vi "Property_Tree Tag_Encode.vi"(7 "Action":T2, 8 "Class":string, 9 "Property Type":T1(ring), 10 "Index":u16, 11 "Method/Property Info":T3) -> (0 "Parents":string[](array[string]), 1 "Indent":i32, 2 "Tag":string, 3 "Bare name":string, 5 "Full name":string)   [LabVIEW 2023]
doc: "By using the long name localized for the tag, children of search matches will be shown. ID is required in tag bc we set the property node terminals by ID.\n\nThe display valule will be the short name for property and method dialogs, and the full name for remove and rearrange dialongs.\n\nFormat is\n\nindex,propertyType,Class,[classID.]ID sting,[class.]parent:shortName \n\nwhere parent:shortName=Long name (localized)\nclass=class of the childmost class in list\nfor dotted properties, the ID string will be of the form classID.propertyID, and the Display name will be of the form Label.Property. \n\nConsider The dotted property Caption.Font. Caption has the class type of Text, so the Class for this tag will be Text, the class ID is 5, and the label contains the Property name \"caption\""
uses:
  controls/action enum.ctl
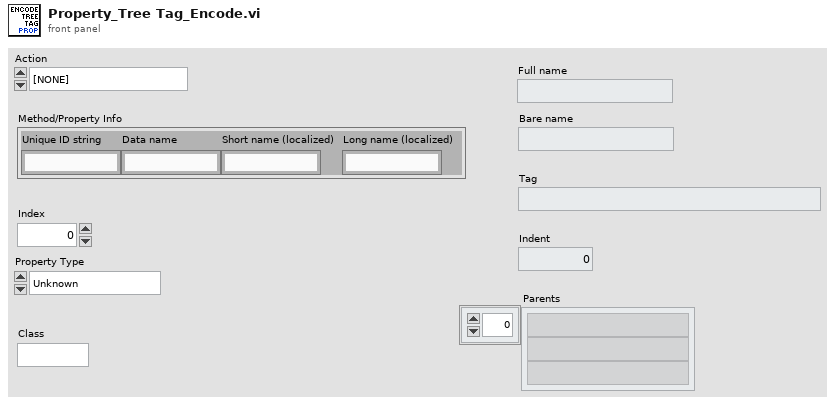
[diagram p1: front panel]
types:
  T1 = enum16{"Unknown", "Base", "Scripting", "Private", "Deprecated", "None", "Divider"}
  T2 = typedef "action enum.ctl" = enum16{"[NONE]", "Wire Bundle", "Wire Unbundle", "Terminal Unbundle", "Terminal Bundle", "Bundler Move Up", "Bundler Move Down", "Bundler Insert", "Bundler Remove", "Bundler Remove Unwired", "Bundler Rearrange", "In Place Insert", "In Place Remove", "In Place Remove Unwired", "In Place Rearrange", "Wire Properties", "Wire Method", "Terminal Properties", "Terminal Method", "Property Move Up", "Property Move Down", "Properties Insert", "Properties Remove", "Properties Remove Unwired", "Properties Rearrange", "Method Change", "Class for Constant", "Class For Control", "Class For Node", "Class Name to Clipboard"}
  T3 = cluster{"Unique ID string":string, "Data name":string, "Short name (localized)":string, "Long name (localized)":string}
  T4 = cluster{"Undotted Property":string, "Bare Property":string, "Is dotted?":bool, "Dot depth":i32, "Indent":i32, "Property Hierarchy":string[], "Parents":string[]}
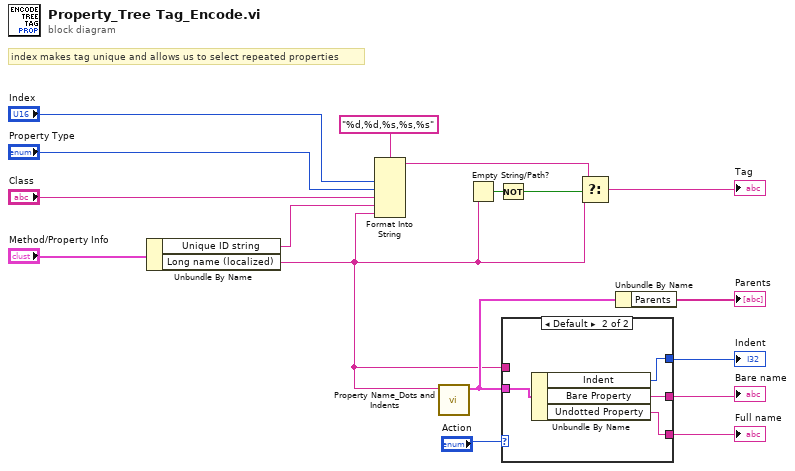
[diagram p0: block diagram]
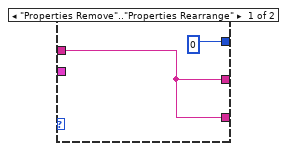
[diagram p2: hidden frame]
diagram:
  # "index makes tag unique and allows us to select repeated properties"
  n1 = Unbundle By Name("Method/Property Info") -> ("Unique ID string"=w15:string, "Long name (localized)"=w2:string)
  n2 = Format Into String(format string="%d,%d,%s,%s,%s", "Index", "Property Type", "Class", w15, w2) -> (resulting string=w14:string)  [unwired: 2 in, 1 out]
  n3 = call "Property Name_Dots and Indents.vi"("Property"=w2) -> ("Cluster"=w4:T4)  [unwired: 10 in]
  n4 = Empty String/Path?(string/path=w2) -> (empty?=w12:bool)
  n5 = Not(x=w12) -> (.not. x?=w11:bool)
  n6 = case shown="Default" "Action" {
    tunnel: [w18 w22] -> w7
    tunnel: w4 -> [_ w23]
    tunnel: [0 w21] -> w5
    tunnel: w2 -> [w18 _]
    tunnel: [w18 w20] -> w1
    frame "Properties Remove".."Properties Rearrange" {
    }
    frame Default {
      n7 = Unbundle By Name(w23) -> ("Indent"=w21:i32, "Bare Property"=w22:string, "Undotted Property"=w20:string)
    }
  }
  "Indent" <- w5
  "Bare name" <- w7
  "Full name" <- w1
  n8 = Select(t=w14, s=w11, f=w2) -> (s? t:f=→"Tag":string)
  n9 = Unbundle By Name(w4) -> ("Parents"=→"Parents":string[])
